vi "niRFUtil MASMT FIR Filter (CDB).vi"(7 "continue?":bool, 8 "error in (no error)":errorcluster, 10 "FIR Coefficients":dbl[](array[numeric]), 11 "X":cdb[](array[numeric])) -> (0 "error out":errorcluster, 3 "Filtered X":cdb[](array[numeric]))   [LabVIEW 2015, in "niRFUtil.lvlib"]
doc: "Filters the input sequence <B>X</B> using the direct-form FIR filter specified by <B>FIR Coefficients</B>."
uses:
  niRFUtil.lvlib
  Utilities/niRFMASMT_FFT.dll
panel:
  out "bWorkH":dbl[](array[numeric])
  out "aWorkH":dbl[](array[numeric])
  out "xWorkH":cdb[](array[numeric])
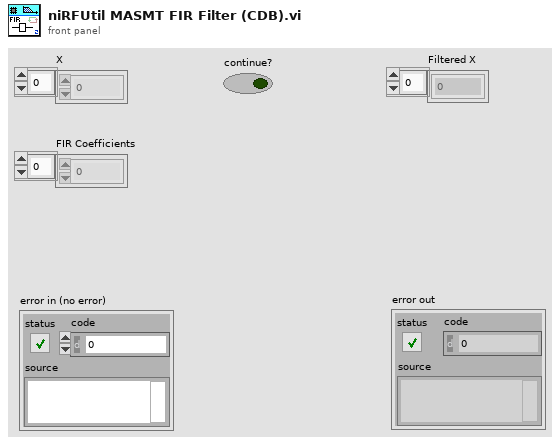
[diagram p1: front panel]
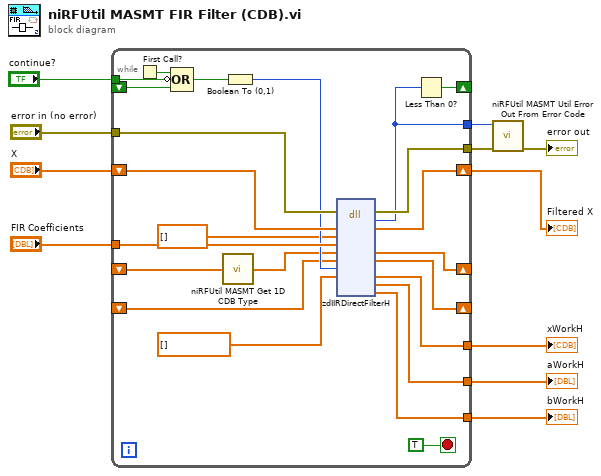
[diagram p0: block diagram]
diagram:
  n1 = while {
    tunnel: "FIR Coefficients" -> [w32]
    tunnel: [w13] -> w2
    tunnel: "error in (no error)" -> [w31]
    tunnel: [w29] -> w7
    tunnel: "continue?" -> [w25]
    tunnel: [w23] -> w5
    tunnel: [w22] -> w4
    shift-right: [w27] -> _
    shift-left: _ -> [w21]
    shift-right: [w17] -> _
    shift-left: _ -> [w19]
    shift-right: [w16] -> _
    shift-left: _ -> [w15]
    tunnel: [w12] -> w1
    shift-right: [w33] -> w10
    shift-left: "X" -> [w34]
    stop <- TRUE stop-if-true
    n2 = First Call?() -> (First Call?: T/F=w26:bool)
    n3 = Compound Arithmetic op=OR(w26, invert w25, w15) -> (w24:bool)
    n4 = call "niRFUtil MASMT Get 1D CDB Type.vi"("1D CDB Array in"=w19) -> ("1D CDB Array out"=w18:cdb[])
    n5 = Boolean To (0,1)(Boolean=w24) -> (0, 1=w30:i16)
    n6 = dll-call lib="C:/Perforce/semoore-sales/Customers/NATI-3813/Noise Floor/LV Filters/ParallelComplexFilterRFUtil/niRFUtil/MASMT/Utilities/niRFMASMT_FFT.*" fn="zdIIRDirectFilterH"(error in=w31, "xH"=w34, "aH"=dbl[] [], "bH"=w32, "x1H"=w18, "y1H"=w21, "reset"=w30, "xWorkH"=cdb[] [] ("Filtered X")) -> (error out=w13:errorcluster, "return type"=w12:i32, "xH"=w33:cdb[], "x1H"=w17:cdb[], "y1H"=w27:dbl[], "xWorkH"=w29:cdb[], "aWorkH"=w23:dbl[], "bWorkH"=w22:dbl[])  [unwired: 7 in, 1 out]
    n7 = Less Than 0?(x=w12) -> (x < 0?=w16:bool)
  }
  "Filtered X" <- w10
  "xWorkH" <- w7
  "aWorkH" <- w5
  "bWorkH" <- w4
  n8 = call "niRFUtil MASMT Util Error Out From Error Code.vi"("error in (no error)"=w2, "error code"=w1) -> ("error out"=→"error out":errorcluster)  [unwired: 9 in]
